vi "Split_path_all.vi"() -> (1 "subdir names":string[](array[string]), 2 "File name":string, 3 "Path array":path[](array[path]), 5 "subdir lengths":i32[](array[numeric]))   [LabVIEW 2012]
panel:
  out "file  exists?":bool
  out "Exists?":bool[](array[boolean])
  in  "Path":path=path "C:/VIs/Files/Split_path_all.vi"
  out "Err?":bool[](array[boolean])
  out "Dir?":bool[](array[boolean])
  out "path types":i16[](array[numeric])
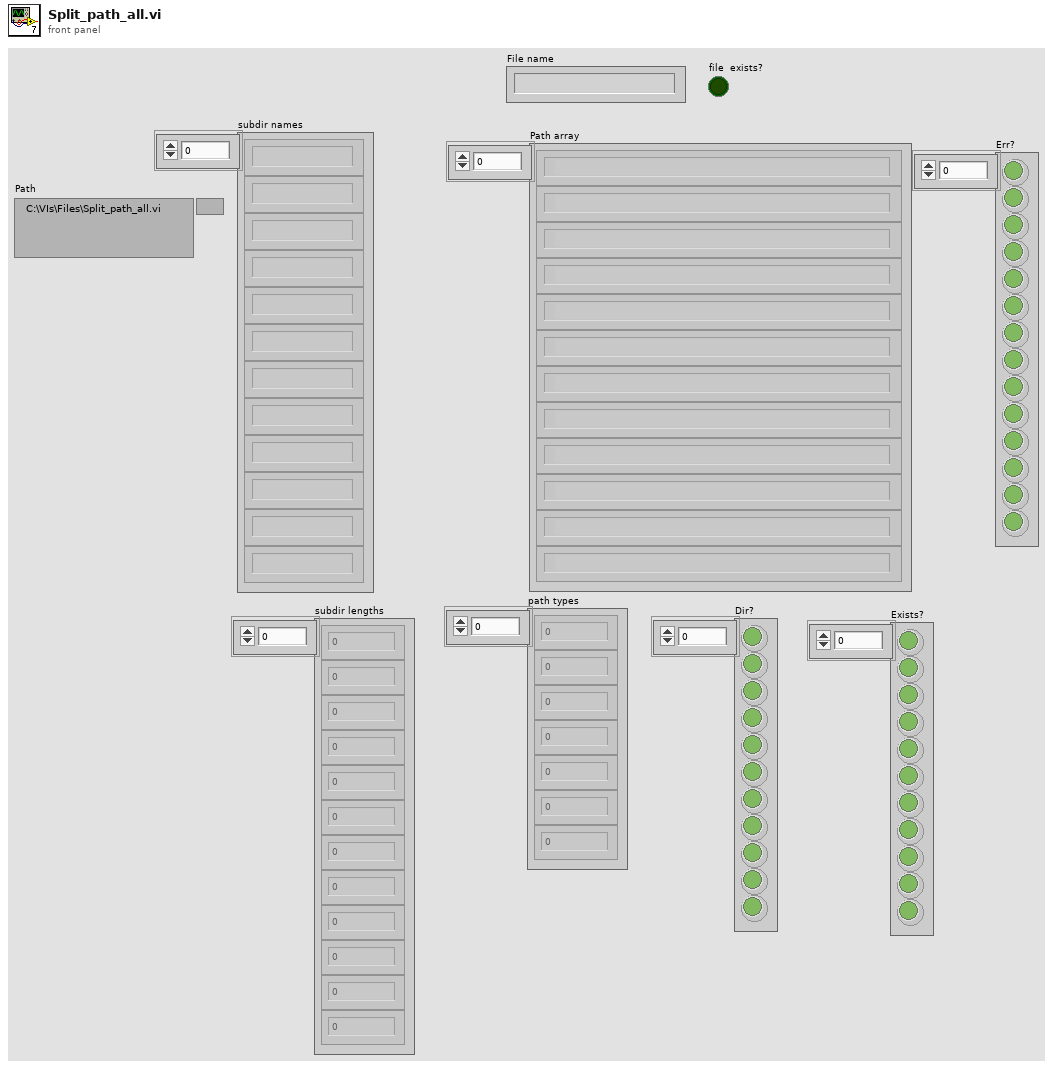
[diagram p1: front panel]
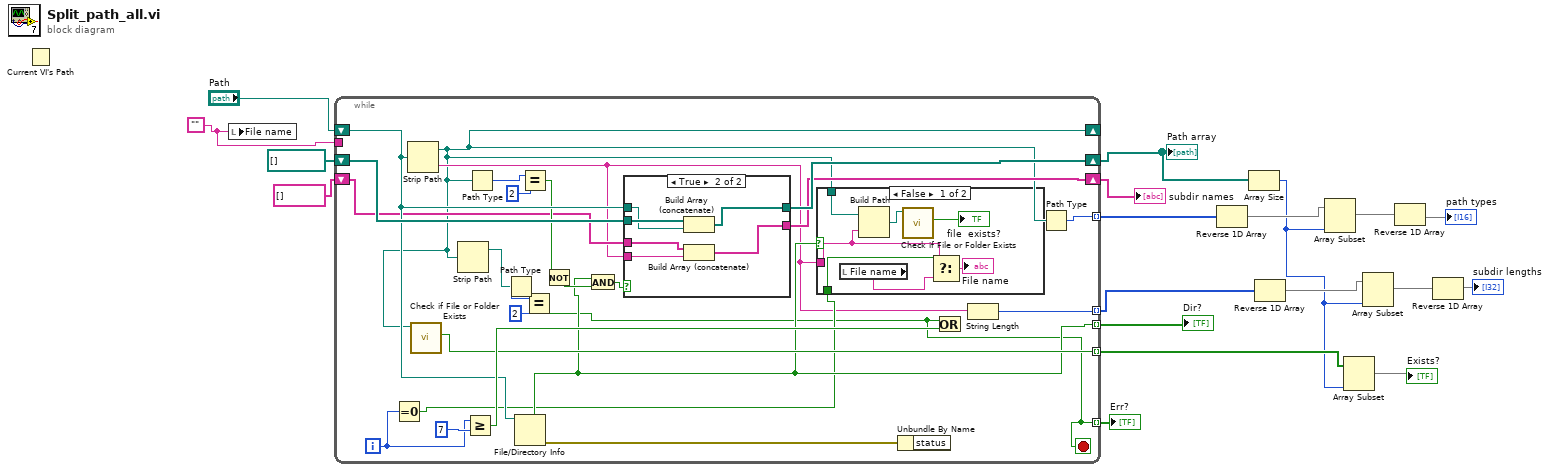
[diagram p0: block diagram]
diagram:
  w13 = ""
  n1 = Current VI's Path() -> ()  [unwired: 1 out]
  n2 = local write "File name"(w13) -> ()
  n3 = while {
    shift-right: [w20] -> _
    shift-left: "Path" -> [w35]
    tunnel: [w42] -> w11 mode=indexing
    tunnel: [w43] -> w5 mode=indexing
    tunnel: [w22] -> w18 mode=indexing
    tunnel: [w28] -> w19 mode=indexing
    tunnel: [w33] -> w3 mode=indexing
    shift-right: [w36] -> w12
    shift-left: path[] [] -> [w37]
    shift-right: [w24] -> w15
    shift-left: string[] [] -> [w25]
    tunnel: w13 -> [_]
    i -> [w27]
    stop <- w22 stop-if-true
    n4 = Equal To 0?(x=w27) -> (x = 0?=w26:bool)
    n5 = Strip Path(path=w35) -> (stripped path=w20:path, name=w23:string)
    n6 = call <vilib>:"Check if File or Folder Exists.vi"("path"=w20) -> ("file or folder exists?"=w33:bool)  [unwired: 8 in, 2 out]
    n7 = Strip Path(path=w20) -> (stripped path=w21:path)  [unwired: 1 out]
    n8 = Greater Or Equal?(x=w27, y=7) -> (x >= y?=w38:bool)
    n9 = Path Type(1:w20) -> (0:w30:i16)
    n10 = Path Type(1:w21) -> (0:w41:i16)
    n11 = File/Directory Info(path=w35) -> (directory=w28:bool, error out=w39:errorcluster)  [unwired: 1 in, 5 out]
    n12 = Equal?(x=w30, y=i16 2) -> (x = y?=w29:bool)
    n13 = Equal?(x=w41, y=i16 2) -> (x = y?=w22:bool)
    n14 = Not(x=w29) -> (.not. x?=w32:bool)
    n15 = And(x=w28, y=w32) -> (x .and. y?=w34:bool)
    n16 = case shown="True" w34 {
      tunnel: w35 -> [_ w58]
      tunnel: [w53 w57] -> w36
      tunnel: w37 -> [w53 w59]
      tunnel: w25 -> [w52 w56]
      tunnel: [w52 w55] -> w24
      tunnel: w23 -> [_ w54]
      frame False {
      }
      frame True {
        n17 = Build Array (concatenate)(w59, w58) -> (w57:path[])
        n18 = Build Array (concatenate)(w56, w54) -> (w55:string[])
      }
    }
    n19 = case shown="False" w28 {
      tunnel: w23 -> [w47 _]
      tunnel: w26 -> [w51 _]
      tunnel: w20 -> [w48 _]
      frame False {
        n20 = local read "File name"() -> (w50:string)
        n21 = Build Path(base path=w48, name or relative path=w47) -> (appended path=w46:path)
        n22 = call <vilib>:"Check if File or Folder Exists.vi"("path"=w46) -> ("file or folder exists?"=→"file  exists?":bool)  [unwired: 8 in, 2 out]
        n23 = Select(t=w47, s=w51, f=w50) -> (s? t:f=→"File name":string)
      }
      frame True {
      }
    }
    n24 = Unbundle By Name(w39) -> ()  [unwired: 1 out]
    n25 = Or(x=w22, y=w38) -> ()  [unwired: 1 out]
    n26 = String Length(string=w23) -> (length=w43:i32)
    n27 = Path Type(1:w20) -> (0:w42:i16)
  }
  "Path array" <- w12
  "subdir names" <- w15
  "Dir?" <- w19
  "Err?" <- w18
  n28 = Reverse 1D Array(array=w11) -> (reversed array=w10:i16[])
  n29 = Array Size(array=w12) -> (size(s)=w2:i32)
  n30 = Reverse 1D Array(array=w5) -> (reversed array=w6:i32[])
  n31 = Array Subset(array=w10, length=w2) -> (w9:i16[])  [unwired: 1 in]
  n32 = Array Subset(array=w3, length=w2) -> (→"Exists?":bool[])  [unwired: 1 in]
  n33 = Array Subset(array=w6, length=w2) -> (w7:i32[])  [unwired: 1 in]
  n34 = Reverse 1D Array(array=w9) -> (reversed array=→"path types":i16[])
  n35 = Reverse 1D Array(array=w7) -> (reversed array=→"subdir lengths":i32[])
